vi "Read Test Log.vi"(8 "error in (no error)":errorcluster, 11 "Post Analysis in":refnum<class "Post Analysis.lvclass">) -> (0 "error out":errorcluster, 2 "Test Log":refnum<vi>, 3 "Post Analysis out":refnum<class "Post Analysis.lvclass">)   [LabVIEW 2023, in "Data Analysis.lvlib" / "Post Analysis.lvlib" / "Post Analysis.lvclass"]
uses:
  Post Analysis.lvclass
  Post Analysis.lvclass/Post Analysis.ctl
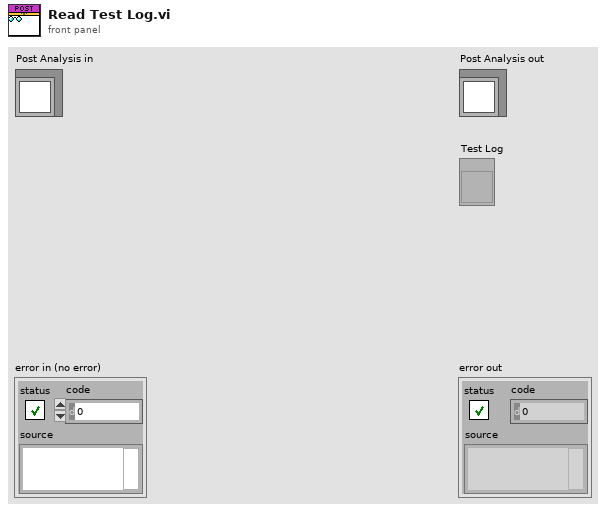
[diagram p1: front panel]
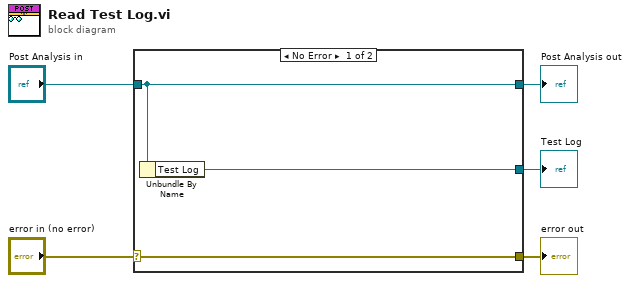
[diagram p0: block diagram]
diagram:
  n1 = case shown="No Error" "error in (no error)" {
    selector: "error in (no error)" -> [w8 w9]
    tunnel: [w8 w9] -> w4
    tunnel: [w7 w10] -> w2
    tunnel: "Post Analysis in" -> [w7 w10]
    tunnel: [w6 _] -> w1
    frame No Error {
      n2 = Unbundle By Name(w7) -> ("Test Log"=w6:refnum<vi>)
    }
    frame Error {
    }
  }
  "error out" <- w4
  "Post Analysis out" <- w2
  "Test Log" <- w1
